vi "删除特大值数据.vi"(2 "数组－数值 2":dbl[](array[numeric]), 3 "数组－数值":dbl[](array[numeric])) -> (0 "数组 6":dbl[](array[numeric]), 1 "数组 5":dbl[](array[numeric]))   [LabVIEW 2016]
panel:
  out "数组 2":dbl[](array[numeric])
  out "数组":dbl[](array[numeric])
  in  "数组 4":dbl[](array[numeric])
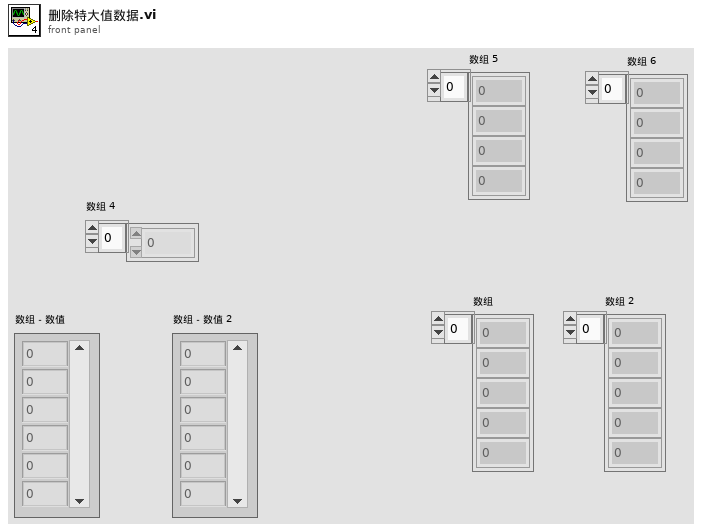
[diagram p1: front panel]
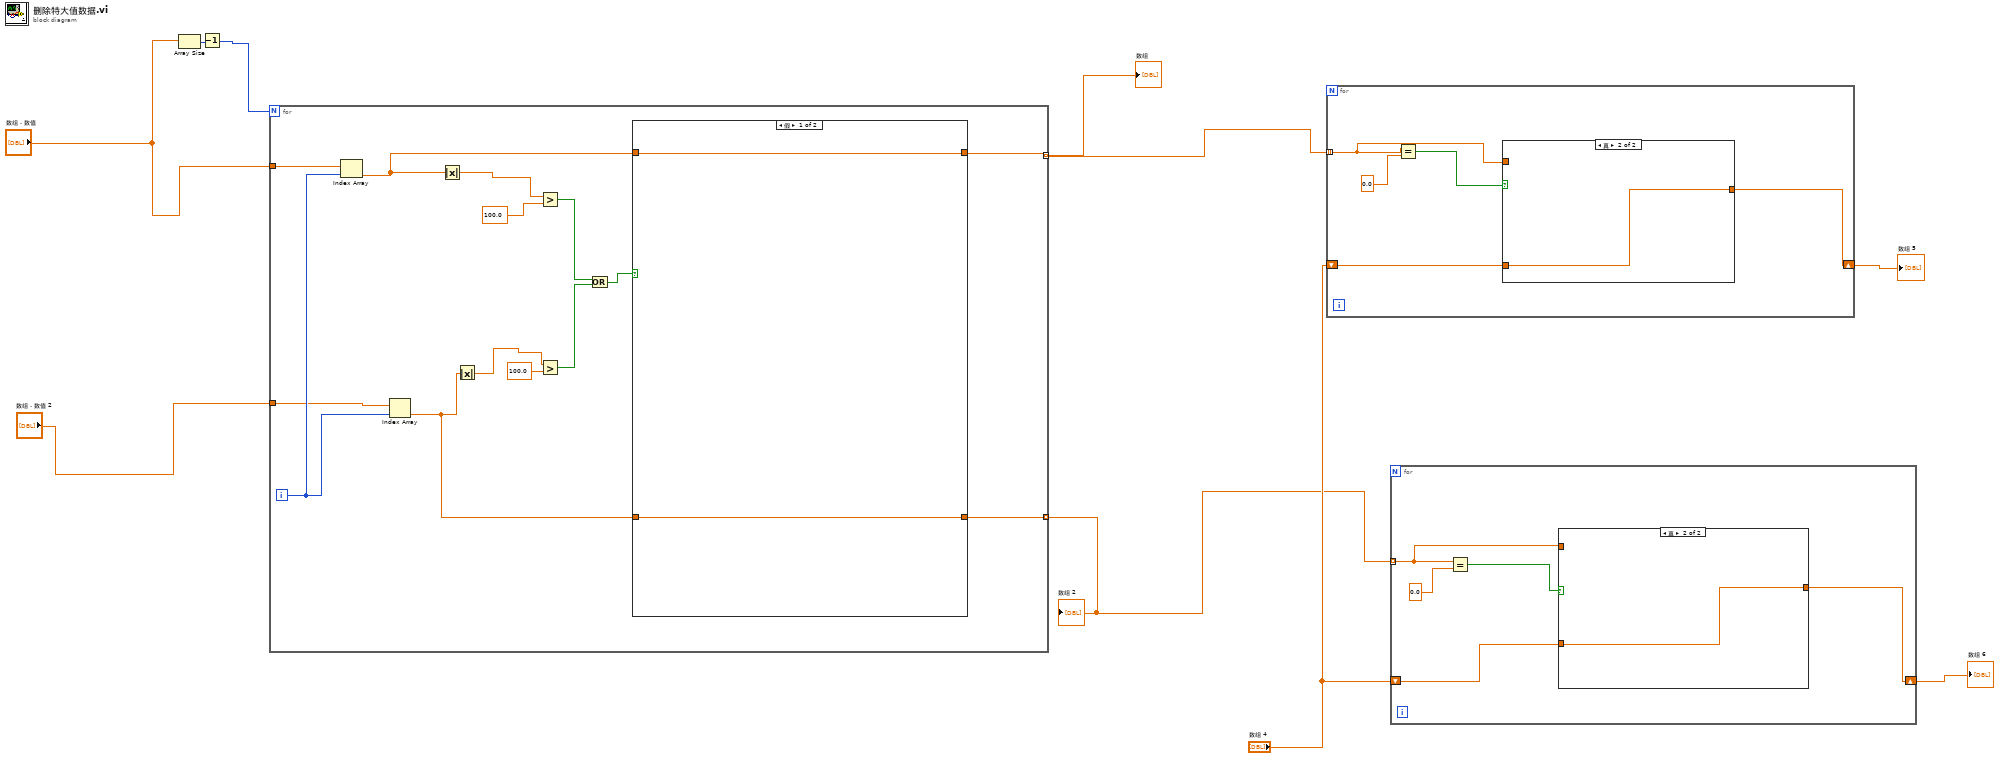
[diagram p0: block diagram]
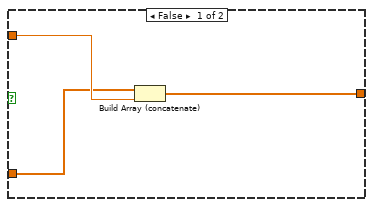
[diagram p3: hidden frame]
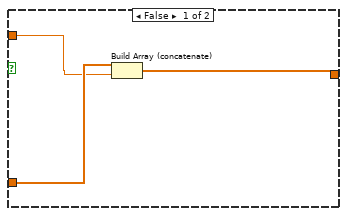
[diagram p4: hidden frame]
diagram:
  n1 = Array Size(array="数组－数值") -> (size(s)=w2:i32)
  n2 = Decrement(x=w2) -> (x-1=w1:i32)
  n3 = for {
    N: w1 -> [_]
    tunnel: "数组－数值" -> [w22]
    tunnel: "数组－数值 2" -> [w21]
    tunnel: [w15] -> w8 mode=indexing
    tunnel: [w14] -> w7 mode=indexing
    i -> [w23]
    n4 = Index Array(array=w22, index=w23) -> (element=w13:dbl)
    n5 = Index Array(array=w21, index=w23) -> (element=w12:dbl)
    n6 = Absolute Value(x=w13) -> (abs(x)=w11:dbl)
    n7 = Absolute Value(x=w12) -> (abs(x)=w10:dbl)
    n8 = Greater?(x=w11, y=100.0) -> (0:w18:bool)
    n9 = Greater?(x=w10, y=100.0) -> (0:w17:bool)
    n10 = Or(x=w18, y=w17) -> (x .or. y?=w16:bool)
    n11 = case shown="假" w16 {
      tunnel: w13 -> [w25 _]
      tunnel: w12 -> [w24 _]
      tunnel: [w25 _] -> w15
      tunnel: [w24 _] -> w14
      frame False {
      }
      frame True {
      }
    }
  }
  "数组" <- w8
  "数组 2" <- w7
  n12 = for {
    tunnel: w8 -> [w28] mode=indexing
    shift-right: [w26] -> w4
    shift-left: "数组 4" -> [w27]
    n13 = Equal?(x=w28, y=0.0) -> (x = y?=w29:bool)
    n14 = case shown="真" w29 {
      tunnel: w28 -> [w31 _]
      tunnel: w27 -> [w32 w34]
      tunnel: [w33 w34] -> w26
      frame False {
        n15 = Build Array (concatenate)(w32, w31) -> (w33:dbl[])
      }
      frame True {
      }
    }
  }
  "数组 5" <- w4
  n16 = for {
    tunnel: w7 -> [w37] mode=indexing
    shift-right: [w35] -> w3
    shift-left: "数组 4" -> [w36]
    n17 = Equal?(x=w37, y=0.0) -> (x = y?=w38:bool)
    n18 = case shown="真" w38 {
      tunnel: w37 -> [w42 _]
      tunnel: w36 -> [w41 w43]
      tunnel: [w40 w43] -> w35
      frame False {
        n19 = Build Array (concatenate)(w41, w42) -> (w40:dbl[])
      }
      frame True {
      }
    }
  }
  "数组 6" <- w3
